vi "client.vi"() -> ()   [LabVIEW 2019]
uses:
  Generated_client/RPC Messages/Greeter_req.ctl
  Generated_client/RPC Messages/Greeter_req_req_oneof/Greeter_req_req_oneof.lvclass
  Generated_client/RPC Messages/Greeter_req_req_oneof/Greeter_req_req_oneof.lvclass/Greeter_req_req_oneof.ctl
  Generated_client/RPC Messages/Greeter_res_res_oneof/Greeter_res_res_oneof.lvclass/Greeter_res_res_oneof.ctl
  Generated_client/Generated_client.lvlib
  Generated_client/RPC Messages/Greeter_res_res_oneof/Greeter_res_res_oneof.lvclass
panel:
  out "res_byte":u8[](array[numeric])
  out "res_string":string
  out "res_bool":bool
  out "res_double":dbl format="%.2f"
  out "res_float":sgl format="%.2f"
  out "res_sfixed64":i64
  out "res_sfixed32":i32
  out "res_fixed64":u64
  out "res_fixed32":u32
  out "res_sint64":i64
  out "res_sint32":i32
  out "res_uint64":u64
  out "res_uint32":u32
  out "res_int64":i64
  out "res_int32":i32
  out "res_latitude":i32
  in  "req_latitude":i32
  in  "req_byte":u8[](array[numeric])
  in  "req_string":string
  in  "req_bool":bool
  in  "req_double":dbl
  in  "req_float":sgl
  in  "req_sfixed64":i64
  in  "req_sfixed32":i32
  in  "req_fixed64":u64
  in  "req_fixed32":u32
  in  "req_sint64":i64
  in  "req_sint32":i32
  in  "req_uint64":u64
  in  "req_unit32":u32
  in  "req_int64":i64
  in  "req_int32":i32
  in  "req_oneof":T1(ring)
  in  "error in":errorcluster
  out "error out":errorcluster
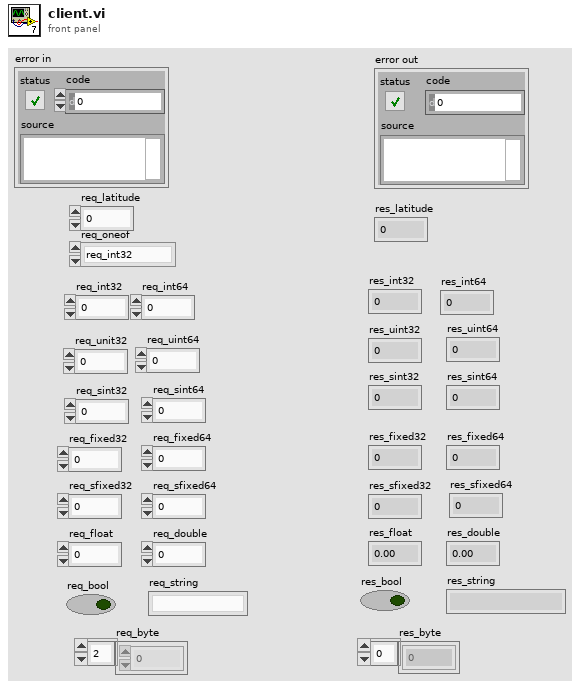
[diagram p1: front panel]
types:
  T1 = enum16{"req_int32", "req_int64", "req_uint32", "req_uint64", "req_sint32", "req_sint64", "req_fixed32", "req_fixed_64", "req_sfixed32", "req_sfixed64", "req_float", "req_double", "req_bool", "req_string", "req_byte"}
  T2 = typedef "Generated_client.lvlib/Greeter_req.ctl" = cluster{"req_latitude":i32, "Greeter_req_req_oneof":refnum<class "Greeter_req_req_oneof.lvclass">}
  T3 = typedef "grpc-lvsupport-release.lvlib/grpcId.ctl" = u64
  T4 = typedef "Generated_client.lvlib/Greeter_res.ctl" = cluster{"res_latitude":i32, "Greeter_res_res_oneof":refnum<class "Greeter_res_res_oneof.lvclass">}
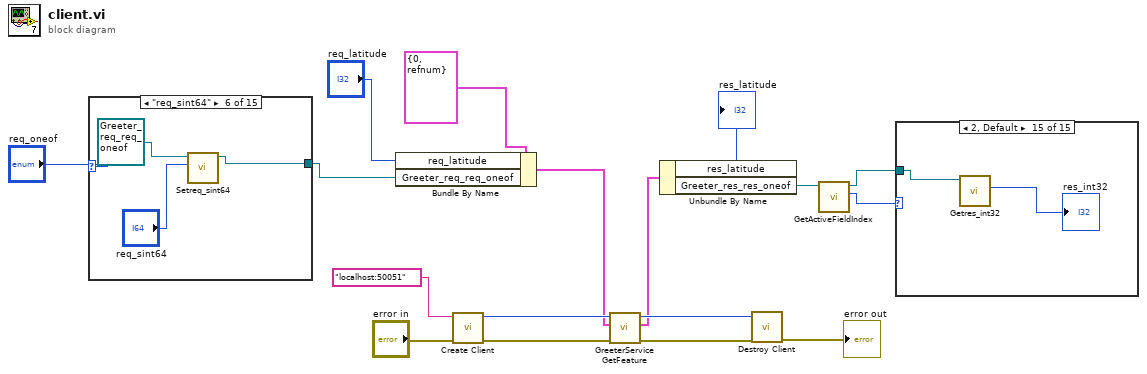
[diagram p0: block diagram]
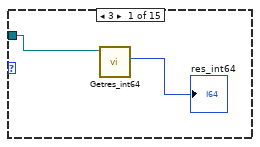
[diagram p2: hidden frame]
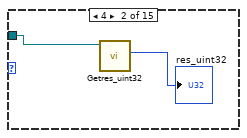
[diagram p3: hidden frame]
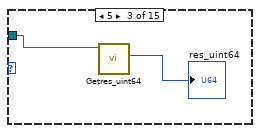
[diagram p4: hidden frame]
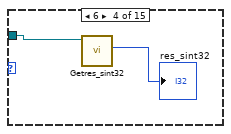
[diagram p5: hidden frame]
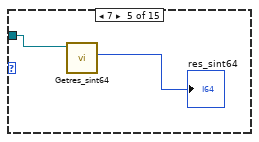
[diagram p6: hidden frame]
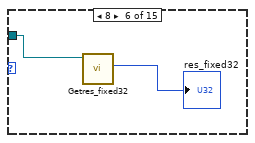
[diagram p7: hidden frame]
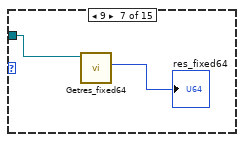
[diagram p8: hidden frame]
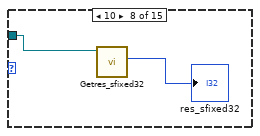
[diagram p9: hidden frame]
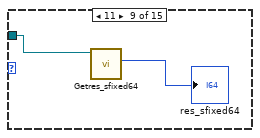
[diagram p10: hidden frame]
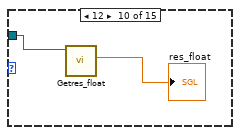
[diagram p11: hidden frame]
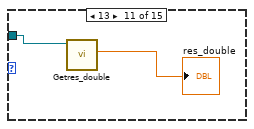
[diagram p12: hidden frame]
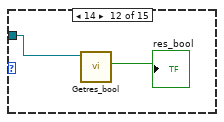
[diagram p13: hidden frame]
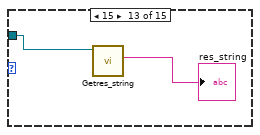
[diagram p14: hidden frame]
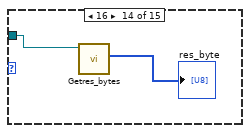
[diagram p15: hidden frame]
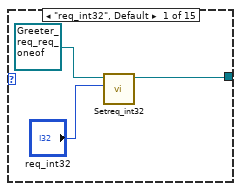
[diagram p16: hidden frame]
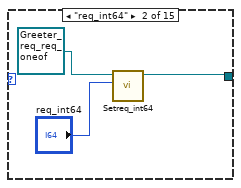
[diagram p17: hidden frame]
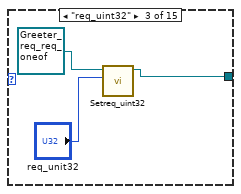
[diagram p18: hidden frame]
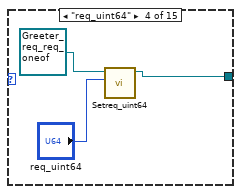
[diagram p19: hidden frame]
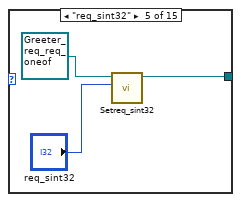
[diagram p20: hidden frame]
diagram:
  n1 = case shown="\"req_sint64\"" "req_oneof" {
    tunnel: [w18 w21 w24 w27 w30 w33 w36 w39 w42 w45 w48 w51 w54 w57 w60] -> w9
    frame "req_int32", Default {
      n2 = call "Setreq_int32.vi"("Set_Val"="req_int32", "OneOfTemplate in"=refnum<class "Greeter_req_req_oneof.lvclass"> refnum) -> ("OneOfTemplate out"=w18:refnum<class "Greeter_req_req_oneof.lvclass">)  [unwired: 8 in, 1 out]
    }
    frame "req_int64" {
      n3 = call "Setreq_int64.vi"("Set_Val"="req_int64", "OneOfTemplate in"=refnum<class "Greeter_req_req_oneof.lvclass"> refnum) -> ("OneOfTemplate out"=w21:refnum<class "Greeter_req_req_oneof.lvclass">)  [unwired: 8 in, 1 out]
    }
    frame "req_uint32" {
      n4 = call "Setreq_uint32.vi"("Set_Val"="req_unit32", "OneOfTemplate in"=refnum<class "Greeter_req_req_oneof.lvclass"> refnum) -> ("OneOfTemplate out"=w24:refnum<class "Greeter_req_req_oneof.lvclass">)  [unwired: 8 in, 1 out]
    }
    frame "req_uint64" {
      n5 = call "Setreq_uint64.vi"("Set_Val"="req_uint64", "OneOfTemplate in"=refnum<class "Greeter_req_req_oneof.lvclass"> refnum) -> ("OneOfTemplate out"=w27:refnum<class "Greeter_req_req_oneof.lvclass">)  [unwired: 8 in, 1 out]
    }
    frame "req_sint32" {
      n6 = call "Setreq_sint32.vi"("Set_Val"="req_sint32", "OneOfTemplate in"=refnum<class "Greeter_req_req_oneof.lvclass"> refnum) -> ("OneOfTemplate out"=w30:refnum<class "Greeter_req_req_oneof.lvclass">)  [unwired: 8 in, 1 out]
    }
    frame "req_sint64" {
      n7 = call "Setreq_sint64.vi"("Set_Val"="req_sint64", "OneOfTemplate in"=refnum<class "Greeter_req_req_oneof.lvclass"> refnum) -> ("OneOfTemplate out"=w33:refnum<class "Greeter_req_req_oneof.lvclass">)  [unwired: 8 in, 1 out]
    }
    frame "req_fixed32" {
      n8 = call "Setreq_fixed32.vi"("Set_Val"="req_fixed32", "OneOfTemplate in"=refnum<class "Greeter_req_req_oneof.lvclass"> refnum) -> ("OneOfTemplate out"=w36:refnum<class "Greeter_req_req_oneof.lvclass">)  [unwired: 8 in, 1 out]
    }
    frame "req_fixed_64" {
      n9 = call "Setreq_fixed64.vi"("Set_Val"="req_fixed64", "OneOfTemplate in"=refnum<class "Greeter_req_req_oneof.lvclass"> refnum) -> ("OneOfTemplate out"=w39:refnum<class "Greeter_req_req_oneof.lvclass">)  [unwired: 8 in, 1 out]
    }
    frame "req_sfixed32" {
      n10 = call "Setreq_sfixed32.vi"("Set_Val"="req_sfixed32", "OneOfTemplate in"=refnum<class "Greeter_req_req_oneof.lvclass"> refnum) -> ("OneOfTemplate out"=w42:refnum<class "Greeter_req_req_oneof.lvclass">)  [unwired: 8 in, 1 out]
    }
    frame "req_sfixed64" {
      n11 = call "Setreq_sfixed64.vi"("Set_Val"="req_sfixed64", "OneOfTemplate in"=refnum<class "Greeter_req_req_oneof.lvclass"> refnum) -> ("OneOfTemplate out"=w45:refnum<class "Greeter_req_req_oneof.lvclass">)  [unwired: 8 in, 1 out]
    }
    frame "req_float" {
      n12 = call "Setreq_float.vi"("Set_Val"="req_float", "OneOfTemplate in"=refnum<class "Greeter_req_req_oneof.lvclass"> refnum) -> ("OneOfTemplate out"=w48:refnum<class "Greeter_req_req_oneof.lvclass">)  [unwired: 8 in, 1 out]
    }
    frame "req_double" {
      n13 = call "Setreq_double.vi"("Set_Val"="req_double", "OneOfTemplate in"=refnum<class "Greeter_req_req_oneof.lvclass"> refnum) -> ("OneOfTemplate out"=w51:refnum<class "Greeter_req_req_oneof.lvclass">)  [unwired: 8 in, 1 out]
    }
    frame "req_bool" {
      n14 = call "Setreq_bool.vi"("Set_Val"="req_bool", "OneOfTemplate in"=refnum<class "Greeter_req_req_oneof.lvclass"> refnum) -> ("OneOfTemplate out"=w54:refnum<class "Greeter_req_req_oneof.lvclass">)  [unwired: 8 in, 1 out]
    }
    frame "req_string" {
      n15 = call "Setreq_string.vi"("Set_Val"="req_string", "OneOfTemplate in"=refnum<class "Greeter_req_req_oneof.lvclass"> refnum) -> ("OneOfTemplate out"=w57:refnum<class "Greeter_req_req_oneof.lvclass">)  [unwired: 8 in, 1 out]
    }
    frame "req_byte" {
      n16 = call "Setreq_bytes.vi"("Set_Val"="req_byte", "OneOfTemplate in"=refnum<class "Greeter_req_req_oneof.lvclass"> refnum) -> ("OneOfTemplate out"=w60:refnum<class "Greeter_req_req_oneof.lvclass">)  [unwired: 8 in, 1 out]
    }
  }
  n17 = Bundle By Name(cluster=T2 {"req_latitude"=0, "Greeter_req_req_oneof"=refnum} ("Greeter_req"), "req_latitude"="req_latitude", "Greeter_req_req_oneof"=w9) -> (w7:T2)
  n18 = call "Create Client.vi"("error in"="error in", "address"="localhost:50051") -> ("error out"=w15:errorcluster, "gRPC ID Out"=w17:T3)  [unwired: 8 in]
  n19 = call "GreeterService GetFeature.vi"("error in"=w15, "Request Data"=w7, "gRPC ID"=w17) -> ("error out"=w14:errorcluster, "Response Data"=w6:T4, "gRPC ID out"=w16:T3)  [unwired: 6 in]
  n20 = Unbundle By Name(w6) -> ("res_latitude"=→"res_latitude":i32, "Greeter_res_res_oneof"=w4:refnum<class "Greeter_res_res_oneof.lvclass">)
  n21 = call "Destroy Client.vi"("error in"=w14, "gRPC ID"=w16) -> ("error out"=→"error out":errorcluster)  [unwired: 9 in]
  n22 = call "GetActiveFieldIndex.vi"("OneOfTemplate in"=w4) -> ("Active Field Index"=w3:i32, "OneOfTemplate out"=w2:refnum<class "Greeter_res_res_oneof.lvclass">)  [unwired: 8 in, 1 out]
  n23 = case shown="2, Default" w3 {
    tunnel: w2 -> [w63 w66 w68 w70 w71 w73 w75 w78 w79 w81 w83 w85 w87 w89 w92]
    frame 3 {
      n24 = call "Getres_int64.vi"("OneOfTemplate in"=w63) -> ("Get_Val"=→"res_int64":i64)  [unwired: 8 in, 2 out]
    }
    frame 4 {
      n25 = call "Getres_uint32.vi"("OneOfTemplate in"=w66) -> ("Get_Val"=→"res_uint32":u32)  [unwired: 8 in, 2 out]
    }
    frame 5 {
      n26 = call "Getres_uint64.vi"("OneOfTemplate in"=w68) -> ("Get_Val"=→"res_uint64":u64)  [unwired: 8 in, 2 out]
    }
    frame 6 {
      n27 = call "Getres_sint32.vi"("OneOfTemplate in"=w70) -> ("Get_Val"=→"res_sint32":i32)  [unwired: 8 in, 2 out]
    }
    frame 7 {
      n28 = call "Getres_sint64.vi"("OneOfTemplate in"=w71) -> ("Get_Val"=→"res_sint64":i64)  [unwired: 8 in, 2 out]
    }
    frame 8 {
      n29 = call "Getres_fixed32.vi"("OneOfTemplate in"=w73) -> ("Get_Val"=→"res_fixed32":u32)  [unwired: 8 in, 2 out]
    }
    frame 9 {
      n30 = call "Getres_fixed64.vi"("OneOfTemplate in"=w75) -> ("Get_Val"=→"res_fixed64":u64)  [unwired: 8 in, 2 out]
    }
    frame 10 {
      n31 = call "Getres_sfixed32.vi"("OneOfTemplate in"=w78) -> ("Get_Val"=→"res_sfixed32":i32)  [unwired: 8 in, 2 out]
    }
    frame 11 {
      n32 = call "Getres_sfixed64.vi"("OneOfTemplate in"=w79) -> ("Get_Val"=→"res_sfixed64":i64)  [unwired: 8 in, 2 out]
    }
    frame 12 {
      n33 = call "Getres_float.vi"("OneOfTemplate in"=w81) -> ("Get_Val"=→"res_float":sgl)  [unwired: 8 in, 2 out]
    }
    frame 13 {
      n34 = call "Getres_double.vi"("OneOfTemplate in"=w83) -> ("Get_Val"=→"res_double":dbl)  [unwired: 8 in, 2 out]
    }
    frame 14 {
      n35 = call "Getres_bool.vi"("OneOfTemplate in"=w85) -> ("Get_Val"=→"res_bool":bool)  [unwired: 8 in, 2 out]
    }
    frame 15 {
      n36 = call "Getres_string.vi"("OneOfTemplate in"=w87) -> ("Get_Val"=→"res_string":string)  [unwired: 8 in, 2 out]
    }
    frame 16 {
      n37 = call "Getres_bytes.vi"("OneOfTemplate in"=w89) -> ("Get_Val"=→"res_byte":u8[])  [unwired: 8 in, 2 out]
    }
    frame 2, Default {
      n38 = call "Getres_int32.vi"("OneOfTemplate in"=w92) -> ("Get_Val"=→"res_int32":i32)  [unwired: 8 in, 2 out]
    }
  }
